vi "parse_expression.vi"(11 "input string":string="(+ hello (/ 2 3 4))") -> (3 "Expression out":T1)   [LabVIEW 2021]
uses:
  Expression.ctl
  ExpressionType.ctl
panel:
  out "Tokens":string[](array[string])
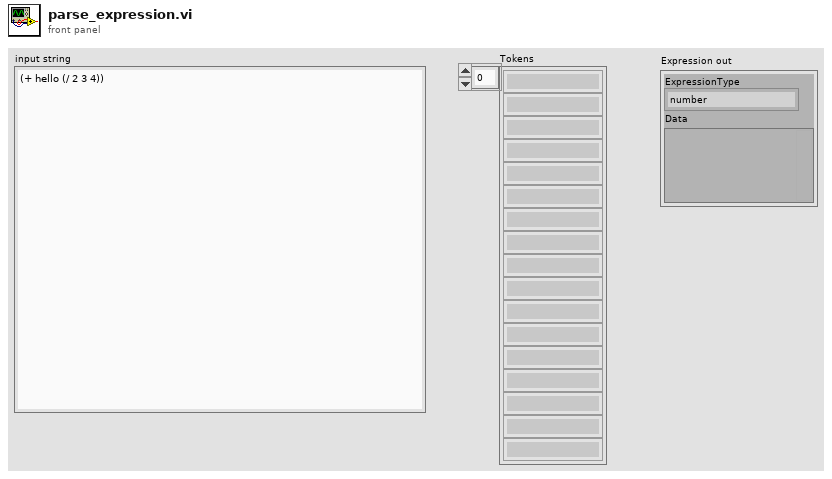
[diagram p1: front panel]
types:
  T1 = typedef "Expression.ctl" = cluster{"ExpressionType":T2, "Data":variant}
  T2 = typedef "ExpressionType.ctl" = enum16{"number", "string", "symbol", "primitive", "list", "closure", "nil", "error"}
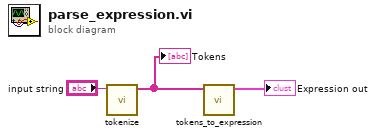
[diagram p0: block diagram]
diagram:
  n1 = call "tokenize.vi"("input string"="input string") -> ("Tokens"=w2:string[])  [unwired: 10 in]
  "Tokens" <- w2
  n2 = call "tokens_to_expression.vi"("Tokens"=w2) -> ("Expression out"=→"Expression out":T1)  [unwired: 10 in]
